vi "MultiChannelfFeedbackCooling (FPGA).vi"() -> ()   [LabVIEW 2013]
doc: "This VI will read single point values from 4 channels of a R Series board at a specified rate."
uses:
  <vilib>/rvi/Emulation/niFpgaSctlEmulationGetInTimedLoop.vi
  <vilib>/rvi/Emulation/niFpgaEmulationReportErrorSimple.vi
  <vilib>/rvi/Emulation/niFpgaGetClockAttributes.vi
  <vilib>/rvi/eio/common/nirviEmuTemplateMethod_errors.vi
  <vilib>/rvi/Memory/Memory_Emulation/nirvimemoryEmulation.vi
  <vilib>/rvi/Memory/Memory_Emulation/nirvimemoryFastEmulation.vi
  <vilib>/rvi/DataTransferAndStorage/Container/Common/niFpgaContainerGetUniqueNameForEmu.vi
  <vilib>/rvi/Memory/Memory_Emulation/niFpgaMemoryEmulationCacheClearOnFirstRun.vi
  <vilib>/rvi/Memory/Memory_Emulation/nirvimemoryEmulationManagerCache_MakeExclusive.vi
  <vilib>/rvi/Memory/Memory_Emulation/niFpgaMemoryEmulationValidateCache.vi
  <vilib>/rvi/Memory/Memory_Emulation/nirvimemoryEmulationManagerCache_ReleaseExclusive.vi
  <vilib>/rvi/Memory/Memory_Emulation/nirvimemoryEmulationManagerCache_InsertValue.vi
  <vilib>/Utility/error.llb/Clear Errors.vi
  <vilib>/rvi/Memory/Memory_Emulation/nirvimemoryEmulationManagerCache_GetValue.vi
  <vilib>/rvi/Memory/Memory_Emulation/nirvimemoryFastEmulationFpgaImpl.vi
  <instcachedir>/0/nirvimemoryFastEmulationFpgaImpl_5FBAB50466BC4C939F684F8805638BFC.lvgen/nirvimemoryFastEmulationFpgaImpl_5FBAB50466BC4C939F684F8805638BFC_003.vi
  <vilib>/rvi/Memory/Memory_Emulation/nirvimemoryEmulationManagerCache_SetValue.vi
  <vilib>/rvi/Emulation/niFpgaSctlEmulationResourceMgr.vi
  <vilib>/rvi/Emulation/niFpgaCriticalErrorInLSC.vi
  <vilib>/rvi/FXPMathLib/FxpInterpret/XNode/nifxpmath_Interpret.xnode
  <vilib>/eio/EIONode/EIONode.xnode
  <vilib>/rvi/DataTransferAndStorage/Container/XNode/niFpgaContainer.xnode
panel:
  out "written_address":u32
  in  "ready_to_write":bool
  in  "Arb steps per cycle":u16
  in  "data_buffer2":i16
  in  "data_buffer_1":i16
  in  "write_address":u16
  in  "meters per measured bit 1":fxp<+/-,16,6>
  in  "meters per measured bit 0":fxp<+/-,16,6>
  in  "apply corrections":bool
  in  "Arb gain (ch2)":fxp<+/-,16,0>=0.4999847412109375 caption="RMS"
  in  "Arb gain (ch1)":fxp<+/-,16,0>=0.4999847412109375 caption="RMS"
  out "fb_1":fxp<+/-,16,16>
  out "fb_0":i16
  out "fb+dc+drive_0":i16
  in  "Zfb norm const":fxp<+/-,16,6>
  in  "meters per bit beam displacement 1":fxp<+/-,16,6>
  in  "Z offset 1":i16
  in  "Drive_gain 1":fxp<+/-,16,0>
  in  "Dc Pos 1":i16
  in  "meters per bit beam displacement 0":fxp<+/-,16,6>
  in  "Dc Pos 0":i16
  in  "Z offset 0":i16
  in  "Zfb norm const 0":fxp<+/-,16,6>
  in  "Drive_gain 0":fxp<+/-,16,0>
  in  "reset freq":bool
  in  "frequency (periods/tick)":fxp<+,32,0>=1.25030055642128e-07
  in  "3, 1":fxp<+/-,16,6>
  in  "3, 2":fxp<+/-,16,6>
  in  "3, 3":fxp<+/-,16,6>
  in  "2, 3":fxp<+/-,16,6>
  in  "2, 2":fxp<+/-,16,6>
  in  "2, 1":fxp<+/-,16,6>
  in  "1, 3":fxp<+/-,16,6>
  in  "1, 2":fxp<+/-,16,6>
  in  "1,1":fxp<+/-,16,6>
  in  "Dc offset 2":i16
  in  "Lower lim 2":fxp<+/-,16,16>
  in  "Upper lim 2":fxp<+/-,16,16>
  in  "dg 2":fxp<+/-,16,12>
  in  "pg 2":fxp<+/-,16,6>
  out "Connector0/AI2":i16
  out "fb +dc_2":i16
  in  "Dc Pos 2":i16
  out "fb+dc+drive_1":i16
  out "Connector0/AI1":i16
  in  "dg 1":fxp<+/-,16,12>
  in  "pg 1":fxp<+/-,16,6>
  in  "Dc offset 1":i16
  in  "Upper lim 1":fxp<+/-,16,16>
  in  "Lower lim 1":fxp<+/-,16,16>
  out "AI0":i16
  in  "dg 0":fxp<+/-,16,12>
  in  "pg 0":fxp<+/-,16,6>
  in  "Dc offset 0":i16
  in  "Upper lim 0":fxp<+/-,16,16>
  in  "Lower lim 0":fxp<+/-,16,16>
  in  "Count(uSec)":u32
  out "FPGA Error Out":errorcluster
  in  "Stop":bool
  # "test"
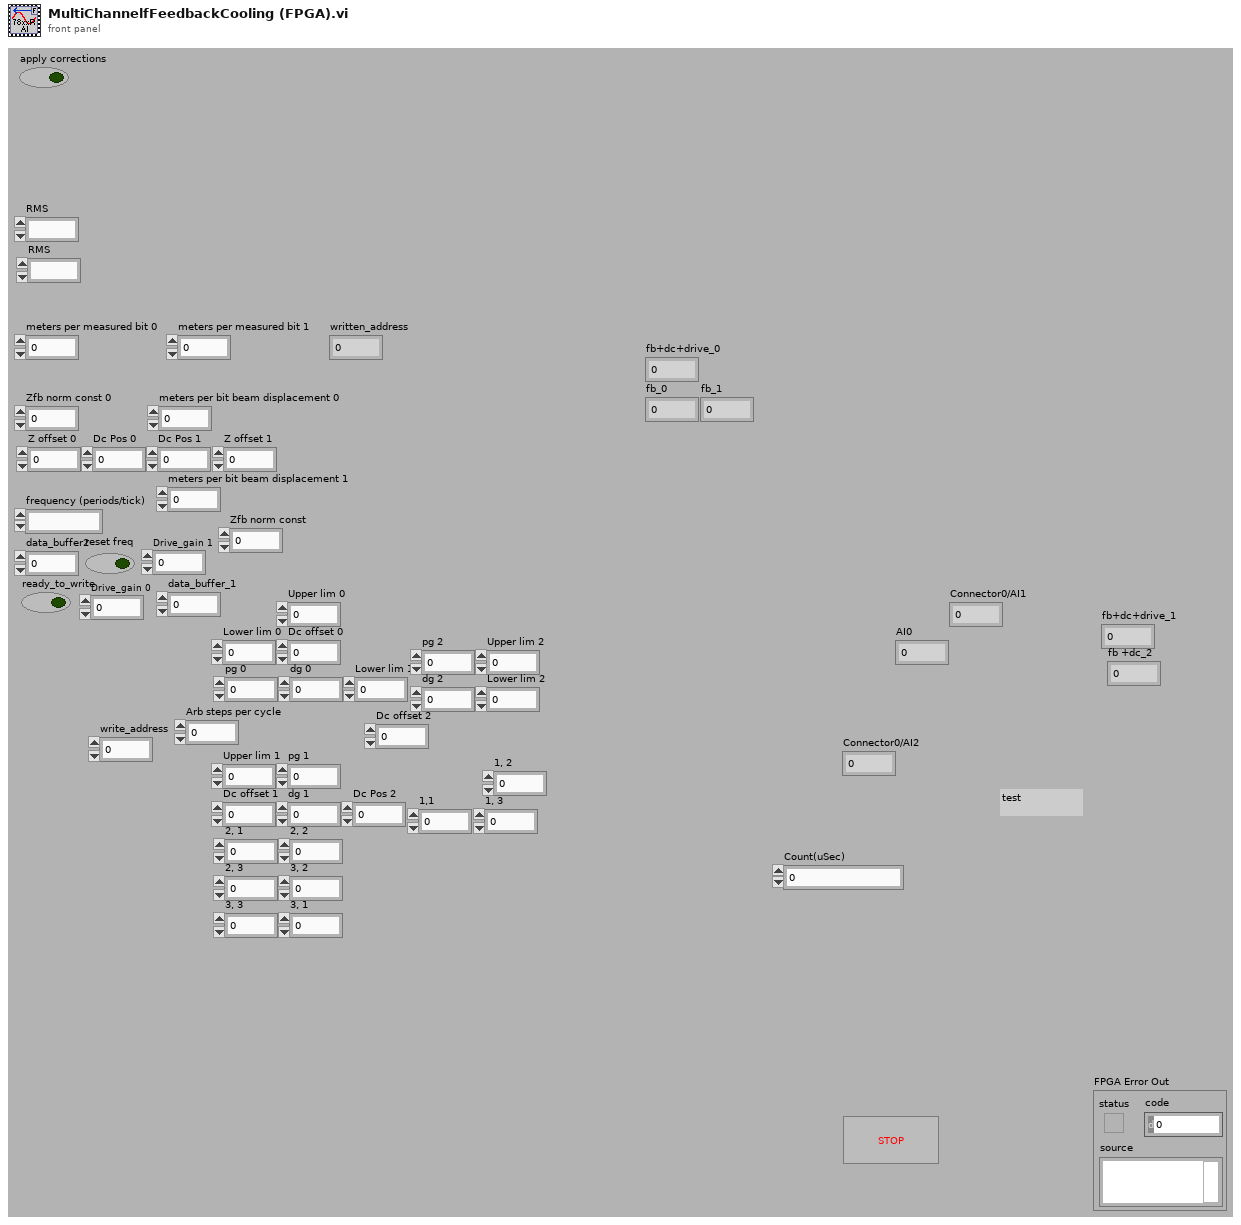
[diagram p1: front panel]
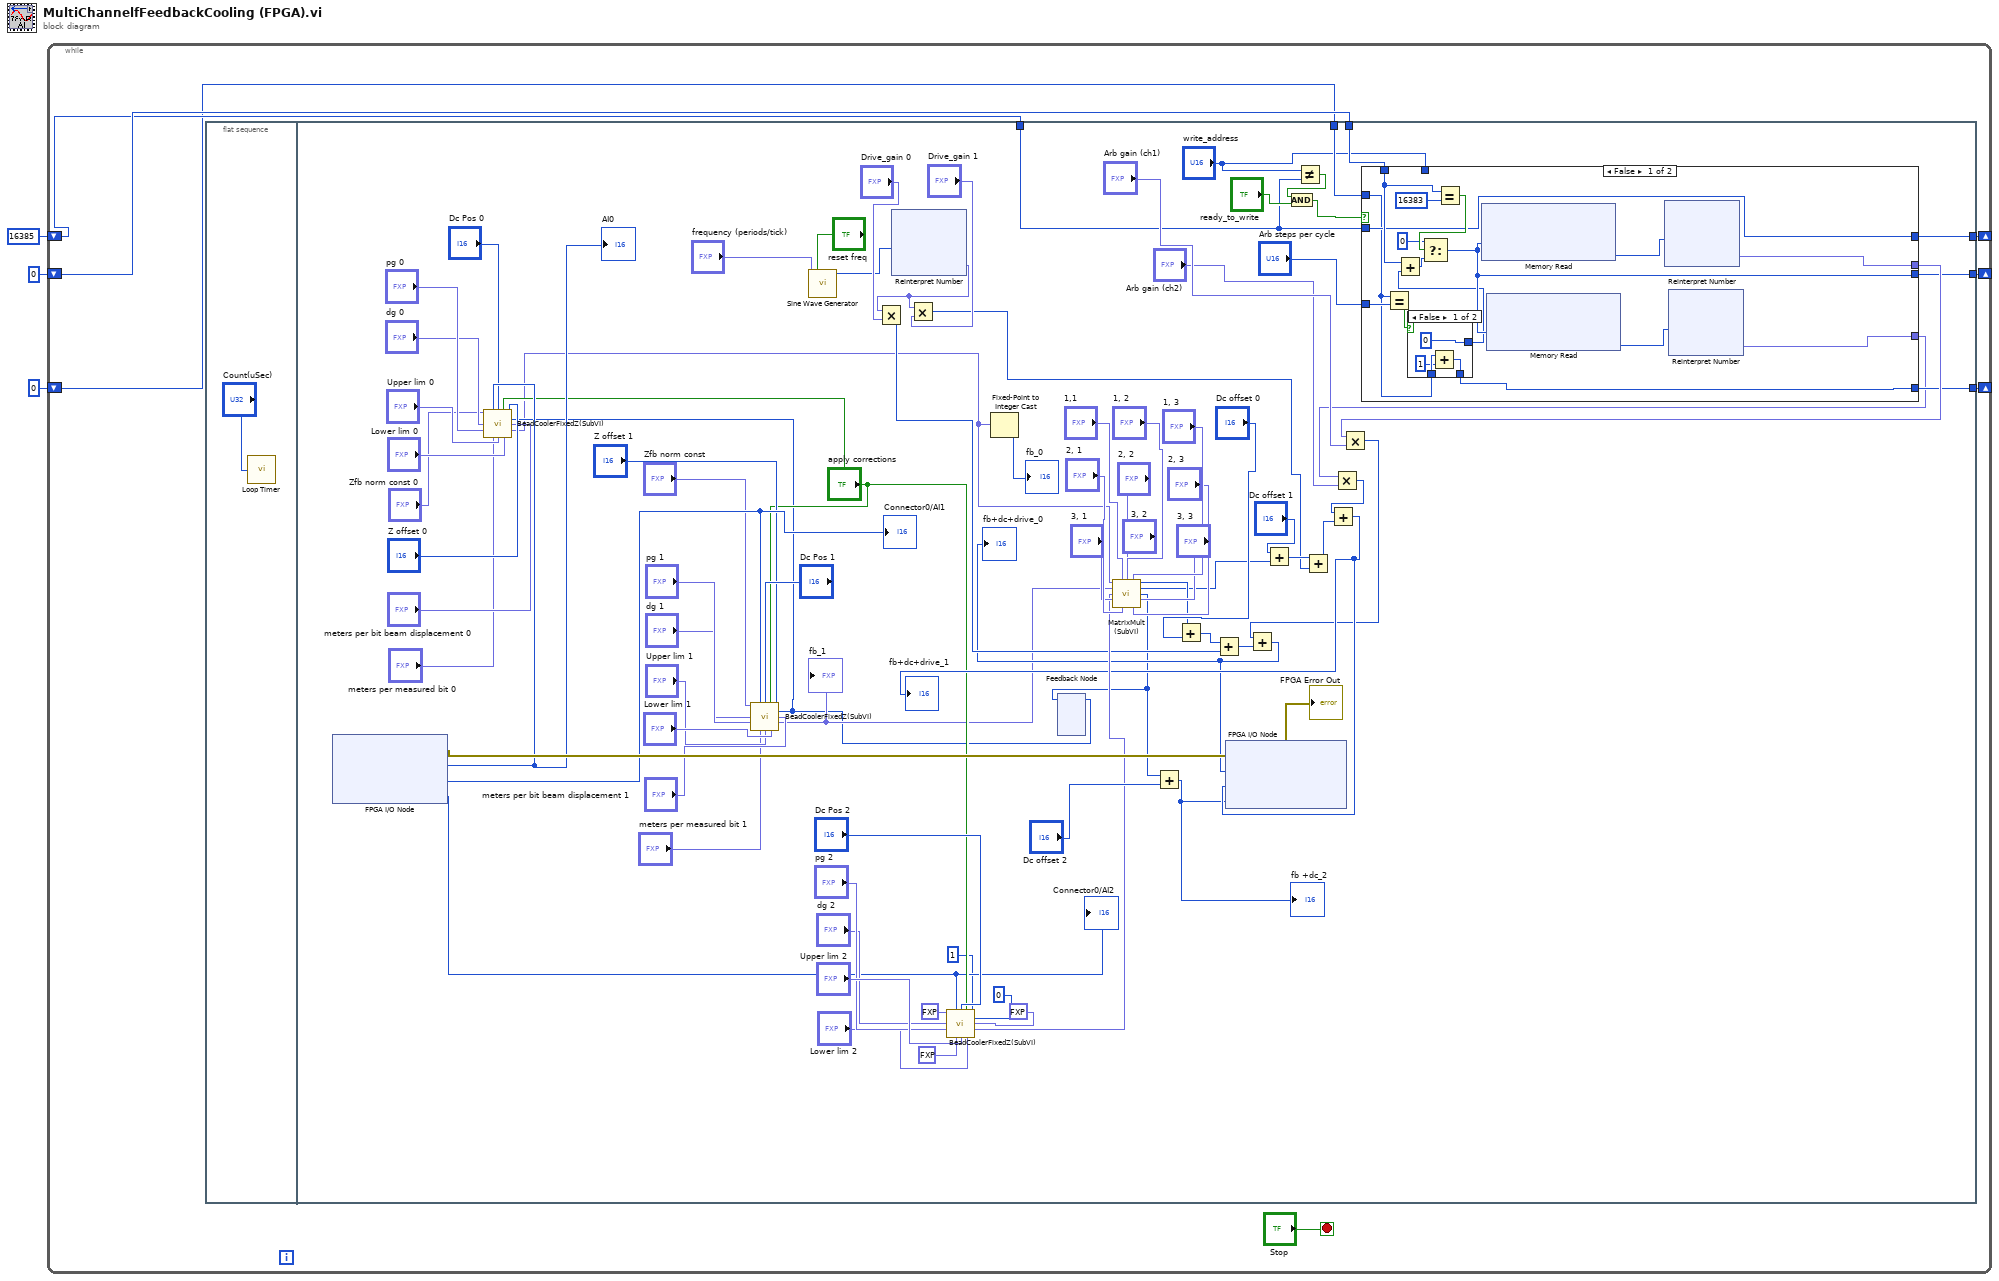
[diagram p0: block diagram]
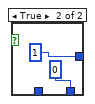
[diagram p2: hidden frame]
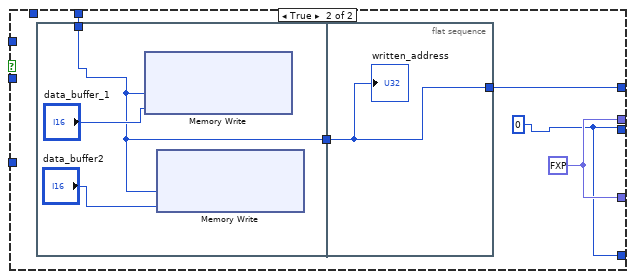
[diagram p3: hidden frame]
diagram:
  n1 = while {
    shift-right: [w9] -> _
    shift-left: u16 0 ("t") -> [w8]
    shift-right: [w7] -> _
    shift-left: u16 0 ("t") -> [w4]
    shift-right: [w6] -> _
    shift-left: u32 16385 ("write_address") -> [w5]
    stop <- "Stop" stop-if-true
    n2 = flat-sequence {
      tunnel: [w34] -> w9
      tunnel: w8 -> [w33]
      tunnel: [w31] -> w7
      tunnel: w4 -> [w30]
      tunnel: [w29] -> w6
      tunnel: w5 -> [w12]
      frame #0 {
        n3 = call "Loop Timer"("Count(uSec)"="Count(uSec)") -> ()  [unwired: 1 out]
      }
      frame #1 {
        n4 = xnode "FPGA I/O Node"() -> ("error out"=w97:errorcluster, "AI0"=w73:i16, "Connector0/AI1"=w68:i16, "Connector0/AI2"=w41:i16)  [unwired: 4 in, 3 out]
        "AI0" <- w73
        "Connector0/AI1" <- w68
        "Connector0/AI2" <- w41
        n5 = call "Sine Wave Generator"("frequency (periods/tick)"="frequency (periods/tick)", "reset"="reset freq") -> ("sine out"=w17:i16)  [unwired: 13 in]
        n6 = xnode "Reinterpret Number"("x"=w17) -> ("y"=w16:fxp<+/-,16,16>)
        n7 = Multiply(x=w16, y="Drive_gain 0") -> (x*y=w53:i16)
        n8 = Multiply(x=w16, y="Drive_gain 1") -> (x*y=w50:i16)
        n9 = call "BeadCoolerFixedZ(SubVI).vi"("Zfb norm const"=fxp<+/-,16,6> 1.0, "AI0"=w41, "Dc Pos"="Dc Pos 2", "apply corrections"="apply corrections", "Z offset"=i16 1, "Z fb"=i16 0, "dg"="dg 2", "meters per bit beam displacement"=fxp<+/-,16,6> 1.0, "pg"="pg 2", "r meters per measured bit"=fxp<+/-,16,6> 1.0, "Upper lim"="Upper lim 2", "Lower lim"="Lower lim 2") -> ("Output"=w58:fxp<+/-,16,16>)  [unwired: 3 in]
        n10 = feedback #1() -> (w42:i16)  [unwired: 1 in]
        n11 = call "BeadCoolerFixedZ(SubVI).vi"("Zfb norm const"="Zfb norm const 0", "AI0"=w73, "Dc Pos"="Dc Pos 0", "apply corrections"="apply corrections", "Z offset"="Z offset 0", "Z fb"=w42, "dg"="dg 0", "meters per bit beam displacement"="meters per bit beam displacement 0", "pg"="pg 0", "r meters per measured bit"="meters per measured bit 0", "Upper lim"="Upper lim 0", "Lower lim"="Lower lim 0") -> ("Output"=w14:fxp<+/-,16,16>)  [unwired: 3 in]
        n12 = call "BeadCoolerFixedZ(SubVI).vi"("Zfb norm const"="Zfb norm const", "AI0"=w68, "Dc Pos"="Dc Pos 1", "apply corrections"="apply corrections", "Z offset"="Z offset 1", "Z fb"=w42, "dg"="dg 1", "meters per bit beam displacement"="meters per bit beam displacement 1", "pg"="pg 1", "r meters per measured bit"="meters per measured bit 1", "Upper lim"="Upper lim 1", "Lower lim"="Lower lim 1") -> ("Output"=w43:fxp<+/-,16,16>)  [unwired: 3 in]
        "fb_1" <- w43
        n13 = Fixed-Point to Integer Cast(1:w14) -> (0:→"fb_0":i16)
        n14 = call "MatrixMult (SubVI).vi"("I"=w14, "1,1"="1,1", "1, 2"="1, 2", "1, 3"="1, 3", "x"=w43, "y"=w58, "3, 1"="3, 1", "3, 3"="3, 3", "3, 2"="3, 2", "2, 1"="2, 1", "2, 2"="2, 2", "2, 3"="2, 3") -> ("v1"=w82:i16, "v2"=w81:i16, "v3"=w44:i16)  [unwired: 1 in]
        n15 = feedback-in #1(w44) -> ()
        n16 = Add(x=w44, y="Dc offset 2") -> (x+y=w40:i16)
        "fb +dc_2" <- w40
        n17 = Add(x=w82, y="Dc offset 0") -> (x+y=w52:i16)
        n18 = Add(x=w52, y=w53) -> (x+y=w48:i16)
        n19 = Add(x="Dc offset 1", y=w81) -> (x+y=w51:i16)
        n20 = Not Equal?(x="write_address", y=w12) -> (x != y?=w26:bool)
        n21 = And(x=w26, y="ready_to_write") -> (x .and. y?=w27:bool)
        n22 = Add(x=w51, y=w50) -> (x+y=w13:i16)
        n23 = case shown="False" w27 {
          tunnel: [w112 w124] -> w37
          tunnel: [w107 w123] -> w34
          tunnel: w33 -> [w104 _]
          tunnel: [w105 w124] -> w22
          tunnel: "Arb steps per cycle" -> [w103 _]
          tunnel: [w98 w123] -> w31
          tunnel: w30 -> [w99 _]
          tunnel: [w102 w121] -> w29
          tunnel: w12 -> [w102 _]
          tunnel: "write_address" -> [_ w120]
          frame False {
            n24 = Equal?(x=w99, y=w103) -> (x = y?=w101:bool)
            n25 = case shown="False" w101 {
              tunnel: [u16 0 ("y") u16 1 ("y")] -> w100
              tunnel: w99 -> [w116 _]
              tunnel: [w114 u16 0] -> w98
              frame False {
                n26 = Add(x=w116, y=u16 1) -> (x+y=w114:u16)
              }
              frame True {
              }
            }
            n27 = Add(x=w104, y=w100) -> (x+y=w108:u16)
            n28 = Equal?(x=w104, y=u16 16383) -> (x = y?=w110:bool)
            n29 = Select(t=u16 0, s=w110, f=w108) -> (s? t:f=w107:u16)
            n30 = xnode ("Memory Read")("Address"=w107) -> ("Data"=w113:i16)  [unwired: 1 in, 1 out]
            n31 = xnode ("Memory Read")("Address"=w107) -> ("Data"=w106:i16)  [unwired: 1 in, 1 out]
            n32 = xnode "Reinterpret Number"("x"=w113) -> ("y"=w112:fxp<+/-,16,16>)
            n33 = xnode "Reinterpret Number"("x"=w106) -> ("y"=w105:fxp<+/-,16,16>)
          }
          frame True {
            w123 = u16 0
            w124 = fxp<+/-,16,16> 0.0 ("y")
            n34 = flat-sequence {
              tunnel: [w125] -> w122
              tunnel: w120 -> [w125]
              tunnel: w122 -> [w128]
              tunnel: [w128] -> w121
              frame #0 {
                n35 = xnode ("Memory Write")("Address"=w125, "Data"="data_buffer_1") -> ()  [unwired: 1 in, 1 out]
                n36 = xnode ("Memory Write")("Address"=w125, "Data"="data_buffer2") -> ()  [unwired: 1 in, 1 out]
              }
              frame #1 {
                "written_address" <- w128
              }
            }
          }
        }
        n37 = Multiply(x=w22, y="Arb gain (ch2)") -> (x*y=w23:i16)
        n38 = Add(x=w23, y=w13) -> (x+y=w49:i16)
        "fb+dc+drive_1" <- w49
        n39 = Multiply(x=w37, y="Arb gain (ch1)") -> (x*y=w35:i16)
        n40 = Add(x=w35, y=w48) -> (x+y=w47:i16)
        "fb+dc+drive_0" <- w47
        n41 = xnode "FPGA I/O Node"("error in"=w97, "Connector0/AO0"=w47, "Connector0/AO1"=w49, "Connector0/AO2"=w40) -> ("error out"=→"FPGA Error Out":errorcluster)  [unwired: 3 in, 3 out]
      }
    }
  }
